vi "Set Shutter Status Extended.vi"(0 "VISA Resource Name":refnum<visa-resource-name>, 5 "Device Number (1)":i32=1, 7 "Shutter Control Number (1)":i32=1, 9 "Shutter Status (0: Open)":enum16{"Open", "Close"}(ring), 11 "error in (no error)":errorcluster {"code" format="%.0x"}) -> (4 "VISA Resource Name Out":refnum<visa-resource-name>, 15 "error out":errorcluster {"code" format="%.0x"})   [LabVIEW 2020, in "Olympus IX BX Series.lvlib"]
doc: "Opens or Closes the shutter.\n\nNotes:\n(1) This VI is valid only for Olympus IX2 model."
uses:
  Olympus IX BX Series.lvlib
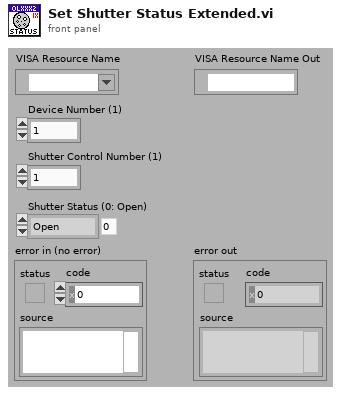
[diagram p1: front panel]
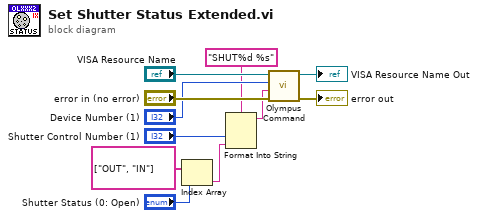
[diagram p0: block diagram]
diagram:
  n1 = Index Array(array=string[] ["OUT", "IN"], index="Shutter Status (0: Open)") -> (element=w1:string)
  n2 = Format Into String(format string="SHUT%d %s", "Shutter Control Number (1)", w1) -> (resulting string=w3:string)  [unwired: 2 in, 1 out]
  n3 = call "Olympus Command.vi"("error in (no error)"="error in (no error)", "Command string"=w3, "Device Number (1)"="Device Number (1)", "VISA Resource Name"="VISA Resource Name") -> ("error out"=→"error out":errorcluster, "VISA Resource Name Out"=→"VISA Resource Name Out":refnum<visa-resource-name>)  [unwired: 5 in, 1 out]
